vi "Get Item IDs By Filter.vi"(8 "error in (no error)":errorcluster, 10 "Table ID":u32=508, 11 "Filter":T1={"Field Name"="Full PN", "Filter Type"="contains", "Filter Value"="80-00000"}) -> (0 "error out":errorcluster, 3 "Item IDs":i32[](array[numeric])=[235])   [LabVIEW 2018]
uses:
  TypeDef/FIlter.ctl
  <vilib>/JDP Science/JSONtext/Next JSON Value.vi
  <vilib>/JDP Science/JSONtext/String Subset.vi
  <vilib>/JDP Science/JSONtext/Parsing/Advance past next JSON Value (inlined COPY).vi
  <vilib>/JDP Science/JSONtext/Parsing/Advance past whitespace.vi
  <vilib>/JDP Science/JSONtext/Parsing/Advance past String.vi
  <vilib>/JDP Science/JSONtext/Parsing/Advance past Number.vi
  <vilib>/JDP Science/JSONtext/Parsing/Advance past Line Ending.vi
  <vilib>/JDP Science/JSONtext/Parsing/Parse Full Path or Item Name.vi
  <vilib>/JDP Science/JSONtext/Parsing/Advance past Array.vi
  <vilib>/JDP Science/JSONtext/Parsing/Advance past Object.vi
  <vilib>/JDP Science/JSONtext/support/Error Cluster From Code.vi
  <vilib>/JDP Science/JSONtext/Offset/Find Item Locations by Path.vi
  <vilib>/JDP Science/JSONtext/JSONtext.lvlib
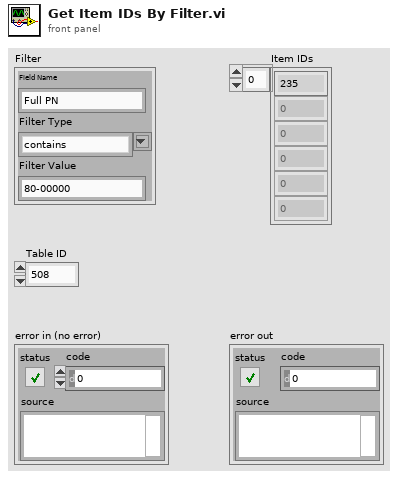
[diagram p1: front panel]
types:
  T1 = typedef "FIlter.ctl" = cluster{"Field Name":string, "Filter Type":string, "Filter Value":string}
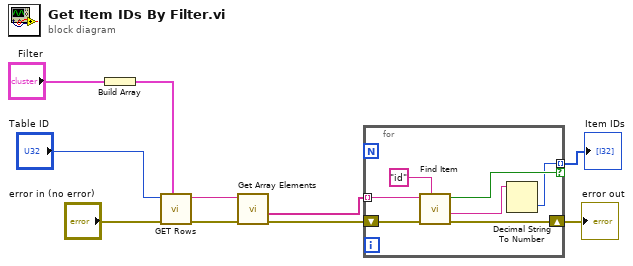
[diagram p0: block diagram]
diagram:
  n1 = Build Array("Filter") -> (w4:T1[])
  n2 = call "GET Rows.vi"("Filters"=w4, "Error in"="error in (no error)", "Table ID"="Table ID") -> ("Error out"=w6:errorcluster, "Rows Array JSON"=w10:string)  [unwired: 7 in]
  n3 = call <vilib>:"Get Array Elements.vi"("error in (no error)"=w6, "JSON"=w10) -> ("error out"=w7:errorcluster, "<JSON>"=w9:string[])  [unwired: 7 in, 1 out]
  n4 = for {
    tunnel: w9 -> [w17] mode=indexing
    shift-right: [w13] -> w5
    shift-left: w7 -> [w14]
    tunnel: [w11] -> w8 mode=indexing if=w15
    n5 = call <vilib>:"Find Item.vi"("$Path or Item Name"="id", "error in (no error)"=w14, "JSON"=w17) -> ("error out"=w13:errorcluster, "<JSON>"=w12:string, "Found"=w15:bool)  [unwired: 5 in, 1 out]
    n6 = Decimal String To Number(string=w12) -> (number=w11:i32)  [unwired: 2 in, 1 out]
  }
  "Item IDs" <- w8
  "error out" <- w5
